vi "Working Shift Change(A-B &C).vi"(0 "From-A":timestamp=timestamp(3526594200 s since 1904-01-01) format="%<%H:%M:%S\n%d/%m/%Y>T", 1 "To-A":timestamp=timestamp(3526451999 s since 1904-01-01) format="%<%H:%M:%S\n%d/%m/%Y>T", 3 "From-B":timestamp=timestamp(3526452000 s since 1904-01-01) format="%<%H:%M:%S\n%d/%m/%Y>T", 4 "To-B":timestamp=timestamp(3526482599 s since 1904-01-01) format="%<%H:%M:%S\n%d/%m/%Y>T", 8 "From-C":timestamp=timestamp(3526482600 s since 1904-01-01) format="%<%H:%M:%S\n%d/%m/%Y>T", 9 "To-C":timestamp=timestamp(3526421399 s since 1904-01-01) format="%<%H:%M:%S\n%d/%m/%Y>T") -> (7 "Shift Change":string="B")   [LabVIEW 2015]
doc: "this vi only used for industial working shifting hour from A to C shift . user can be set the shift time from A to C."
panel:
  out "number 7":i32
  out "number 6":i32
  out "number 5":i32
  out "number 4":i32
  out "number 3":i32
  out "number 2":i32
  out "number":i32
  out "current time":timestamp=timestamp(3539584812.8455925 s since 1904-01-01)
  out "Shift change":u8=2
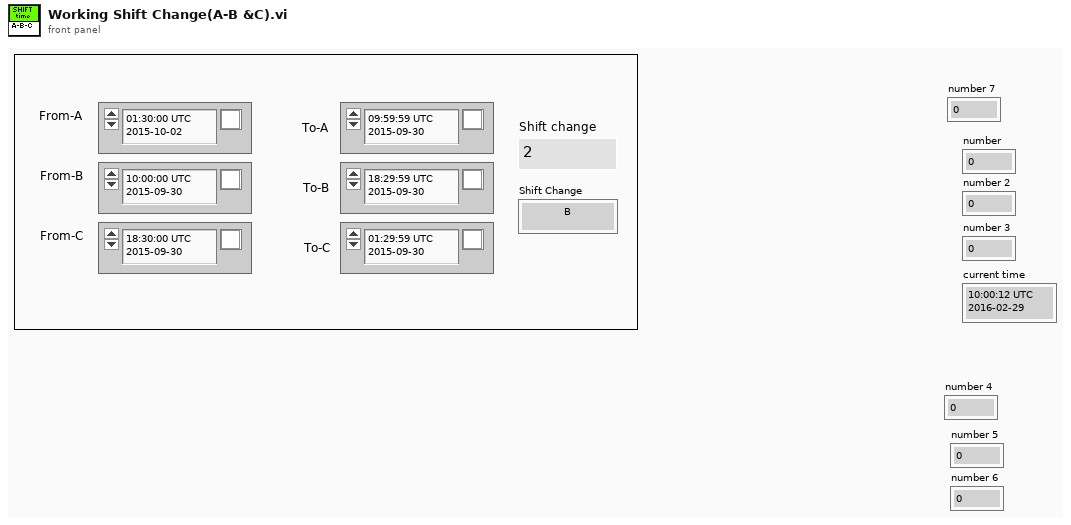
[diagram p1: front panel]
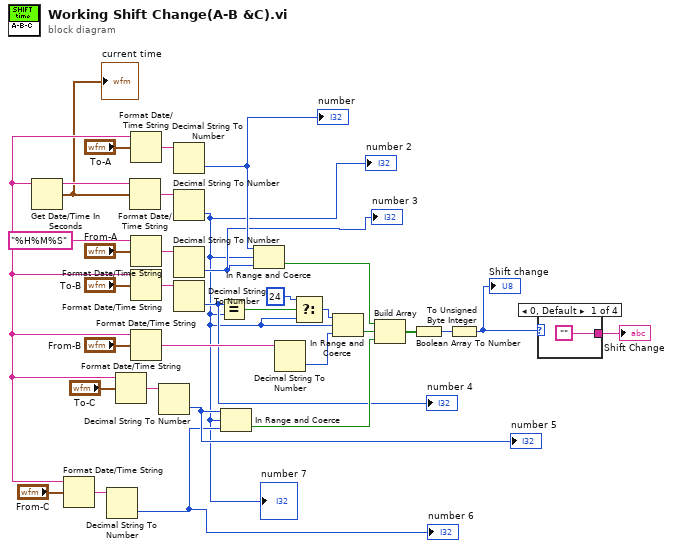
[diagram p0: block diagram]
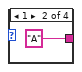
[diagram p2: hidden frame]
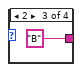
[diagram p3: hidden frame]
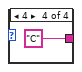
[diagram p4: hidden frame]
diagram:
  w15 = "%H%M%S" ("time format string (%c)")
  n1 = Get Date/Time In Seconds() -> (seconds since 1Jan1904=w14:timestamp)
  "current time" <- w14
  n2 = Format Date/Time String(time format string (%c)=w15, seconds (now)="From-C") -> (date/time string=w22:string)  [unwired: 1 in]
  n3 = Decimal String To Number(string=w22) -> (number=w2:i32)  [unwired: 2 in, 1 out]
  "number 6" <- w2
  n4 = Format Date/Time String(time format string (%c)=w15, seconds (now)="To-C") -> (date/time string=w21:string)  [unwired: 1 in]
  n5 = Format Date/Time String(time format string (%c)=w15, seconds (now)=w14) -> (date/time string=w30:string)  [unwired: 1 in]
  n6 = Format Date/Time String(time format string (%c)=w15, seconds (now)="To-A") -> (date/time string=w29:string)  [unwired: 1 in]
  n7 = Format Date/Time String(time format string (%c)=w15, seconds (now)="From-A") -> (date/time string=w32:string)  [unwired: 1 in]
  n8 = Format Date/Time String(time format string (%c)=w15, seconds (now)="To-B") -> (date/time string=w27:string)  [unwired: 1 in]
  n9 = Format Date/Time String(time format string (%c)=w15, seconds (now)="From-B") -> (date/time string=w26:string)  [unwired: 1 in]
  n10 = Decimal String To Number(string=w21) -> (number=w3:i32)  [unwired: 2 in, 1 out]
  "number 5" <- w3
  n11 = Decimal String To Number(string=w29) -> (number=w6:i32)  [unwired: 2 in, 1 out]
  "number" <- w6
  n12 = Decimal String To Number(string=w30) -> (number=w1:i32)  [unwired: 2 in, 1 out]
  "number 2" <- w1
  "number 7" <- w1
  n13 = Decimal String To Number(string=w32) -> (number=w5:i32)  [unwired: 2 in, 1 out]
  "number 3" <- w5
  n14 = Decimal String To Number(string=w27) -> (number=w4:i32)  [unwired: 2 in, 1 out]
  "number 4" <- w4
  n15 = Equal?(x=w4, y=w1) -> (x = y?=w18:bool)
  n16 = In Range and Coerce(upper limit=w3, x=w1, lower limit=w2) -> (In Range?=w11:bool)  [unwired: 1 out]
  n17 = In Range and Coerce(upper limit=w6, x=w1, lower limit=w5) -> (In Range?=w13:bool)  [unwired: 1 out]
  n18 = Decimal String To Number(string=w26) -> (number=w23:i32)  [unwired: 2 in, 1 out]
  n19 = Select(t=24, s=w18, f=w1) -> (s? t:f=w16:i32)
  n20 = In Range and Coerce(upper limit=w16, x=w1, lower limit=w23) -> (In Range?=w12:bool)  [unwired: 1 out]
  n21 = Build Array(w13, w12, w11) -> (w10:bool[])
  n22 = Boolean Array To Number(Boolean array=w10) -> (number=w9:u32)
  n23 = To Unsigned Byte Integer(number=w9) -> (unsigned 8bit integer=w8:u8)
  "Shift change" <- w8
  n24 = case shown="0, Default" w8 {
    tunnel: ["" "A" "B" "C"] -> w7
    frame 0, Default {
    }
    frame 1 {
    }
    frame 2 {
    }
    frame 4 {
    }
  }
  "Shift Change" <- w7
